vi "CLSUIP_CopyFrontPanelAndConPane.vi"(10 "New VI":refnum<vi>, 11 "Orig VI":refnum<vi>) -> (3 "New VI out":refnum<vi>)   [LabVIEW 2021, in "MemberVICreation.lvlib" / "VIRetooler.lvclass"]
uses:
  <resource>/Framework/Providers/LVClassLibrary/NewAccessors/VIRetooler/VIRetooler.lvclass
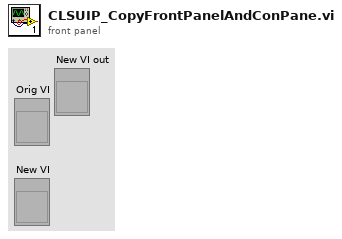
[diagram p1: front panel]
types:
  T1 = typedef "LVPositionTypeDef.ctl" = cluster{"Left":i32, "Top":i32}
  T2 = enum16{"Invalid Wire Rule", "Required", "Recommended", "Optional", "Dynamic Dispatch"}[]
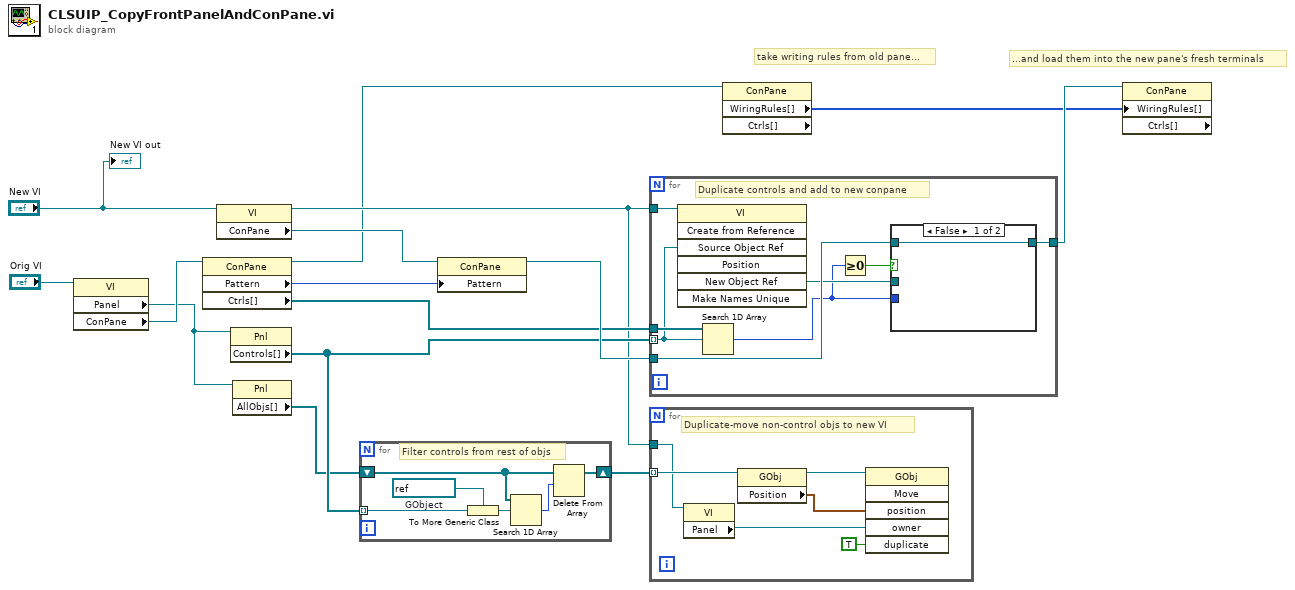
[diagram p0: block diagram]
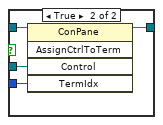
[diagram p2: hidden frame]
diagram:
  # "...and load them into the new pane's fresh terminals"
  # "take writing rules from old pane..."
  n1 = property class="VI"(reference="Orig VI") -> ("Panel"=w8:refnum<vi>, "ConPane"=w12:refnum<vi>)  [unwired: 1 in, 2 out]
  n2 = property class="ConPane"(reference=w12) -> (reference out=w3:refnum<vi>, "Pattern"=w13:u32, "Ctrls[]"=w14:refnum<vi>[])  [unwired: 1 in, 1 out]
  n3 = property class="VI"(reference="New VI") -> (reference out=w4:refnum<vi>, "ConPane"=w11:refnum<vi>)  [unwired: 1 in, 1 out]
  n4 = property class="Pnl"(reference=w8) -> ("Controls[]"=w7:refnum<vi>[])  [unwired: 1 in, 2 out]
  n5 = property class="Pnl"(reference=w8) -> ("AllObjs[]"=w6:refnum<vi>[])  [unwired: 1 in, 2 out]
  n6 = for {
    tunnel: w7 -> [w21] mode=indexing
    shift-right: [w17] -> w5
    shift-left: w6 -> [w18]
    w16 = refnum<vi> refnum  # GObject
    # "Filter controls from rest of objs"
    n7 = To More Generic Class(target class=w16, reference=w21) -> (generic class reference=w20:refnum<vi>)
    n8 = Search 1D Array(1D array=w18, element=w20) -> (index of element=w19:i32)  [unwired: 1 in]
    n9 = Delete From Array(array=w18, length=w19) -> (array with subset deleted=w17:refnum<vi>[])  [unwired: 1 in, 1 out]
  }
  n10 = property class="ConPane"(reference=w11, "Pattern"=w13) -> (reference out=w15:refnum<vi>)  [unwired: 1 in, 1 out]
  n11 = for {
    tunnel: w4 -> [w26]
    tunnel: w7 -> [w23] mode=indexing
    tunnel: w14 -> [w29]
    tunnel: w15 -> [w28]
    tunnel: [w22] -> w2
    # "Duplicate controls and add to new conpane"
    n12 = invoke class="VI" method="Create from Reference"(reference=w26, "Source Object Ref"=w23) -> ("New Object Ref"=w27:refnum<vi>)  [unwired: 5 in, 6 out]
    n13 = Search 1D Array(1D array=w29, element=w23) -> (index of element=w24:i32)  [unwired: 1 in]
    n14 = Greater Or Equal To 0?(x=w24) -> (x >= 0?=w25:bool)
    n15 = case shown="False" w25 {
      tunnel: w28 -> [w30 w34]
      tunnel: w27 -> [_ w33]
      tunnel: w24 -> [_ w32]
      tunnel: [w30 w31] -> w22
      frame False {
      }
      frame True {
        n16 = invoke class="ConPane" method="AssignCtrlToTerm"(reference=w34, "Control"=w33, "TermIdx"=w32) -> (reference out=w31:refnum<vi>)  [unwired: 2 in, 4 out]
      }
    }
  }
  n17 = for {
    tunnel: w5 -> [w36] mode=indexing
    tunnel: w4 -> [w35]
    # "Duplicate-move non-control objs to new VI"
    n18 = property class="VI"(reference=w35) -> ("Panel"=w37:refnum<vi>)  [unwired: 1 in, 2 out]
    n19 = property class="GObj"(reference=w36) -> (reference out=w40:refnum<vi>, "Position"=w39:T1)  [unwired: 1 in, 1 out]
    n20 = invoke class="GObj" method="Move"(reference=w40, "position"=w39, "owner"=w37, "duplicate"=TRUE ("Duplicate? (F)")) -> ()  [unwired: 2 in, 6 out]
  }
  n21 = property class="ConPane" props=["WiringRules[]", "Ctrls[]"](reference=w3) -> ("WiringRules[]"=w1:T2)  [unwired: 1 in, 3 out]
  n22 = property class="ConPane" props=["WiringRules[]", "Ctrls[]"](reference=w2, "WiringRules[]"=w1) -> ()  [unwired: 1 in, 3 out]
  "New VI out" <- "New VI"
